vi "Set_CTRE_Status_Period.vi"(8 "error in (no error)":errorcluster, 10 "Input":T2 {"Frame" items=["Status_1_General"=5120, "Status_2_Feedback0"=5184, "Status_3_Quadrature"=5248, "Status_4_AinTempVbat"=5312, "Status_6_Misc"=5440, "Status_7_CommStatus"=5504, "Status_8_PulseWidth"=5568, "Status_9_MotProfBuffer"=5632, "Status_10_MotionMagic"=5696, "Status_11_UartGadgeteer"=5760, "Status_12_Feedback1"=5824, "Status_13_Base_PIDF0"=5888, "Status_14_Turn_PIDF1"=5952, "Status_15_FirmwareApiStatus"=6016, "Status_Brushless_Current"=4672]}, 11 "PhoenixMotorControlDevRef":T3={"DeviceStatus"={"status"=FALSE, "code"=0, "source"=""}, "Type"=enum."PWM", "PWM"={"PWM Channel"=enum."PWM 1", "DeadBand"={"Name"="", "maxPositivePwm"=0, "minPositivePwm"=0, "centerPwm"=0, "maxNegativePwm"=0, "minNegativePwm"=0, "angularRange"=0}}, "CAN"={"Device Number"=0, "SetOutput VI Ref"=variant(enum8{"Percent VBus", "Current", "Speed", "Position", "Voltage"} enum."Percent VBus"), "GetOutput VI Ref"=variant(refnum<k1> refnum), "Enable VI Ref"=variant(dbl 12.0), "Disable VI Ref"=variant(enum8{"Percent VBus", "Speed", "Position", "Slave", "Unchanged / Invalid", "Voltage Compensation", "Current", "Motion Profile"} enum."Percent VBus"), "Data"=variant}, "Invert"=FALSE, "DIO PWM"={"PWM \"Enable\" Channel"=enum."Invalid", "DIOChannel"=enum."Invalid", "PWM Rate"=0.0}}) -> (0 "error out":errorcluster, 3 "PhoenixMotorControlDevRef 2":T3={"DeviceStatus"={"status"=FALSE, "code"=0, "source"=""}, "Type"=enum."PWM", "PWM"={"PWM Channel"=enum."PWM 1", "DeadBand"={"Name"="", "maxPositivePwm"=0, "minPositivePwm"=0, "centerPwm"=0, "maxNegativePwm"=0, "minNegativePwm"=0, "angularRange"=0}}, "CAN"={"Device Number"=0, "SetOutput VI Ref"=variant(enum8{"Percent VBus", "Current", "Speed", "Position", "Voltage"} enum."Percent VBus"), "GetOutput VI Ref"=variant(refnum<k1> refnum), "Enable VI Ref"=variant(dbl 12.0), "Disable VI Ref"=variant(enum8{"Percent VBus", "Speed", "Position", "Slave", "Unchanged / Invalid", "Voltage Compensation", "Current", "Motion Profile"} enum."Percent VBus"), "Data"=variant}, "Invert"=FALSE, "DIO PWM"={"PWM \"Enable\" Channel"=enum."Invalid", "DIOChannel"=enum."Invalid", "PWM Rate"=0.0}})   [LabVIEW 2020]
uses:
  <vilib>/Rock Robotics/WPI/MotorControl/WPI_MotorControlDeviceRef.ctl
  <vilib>/Rock Robotics/WPI/MotorControl/WPI_MotorControlType.ctl
  <vilib>/Rock Robotics/SystemInterfaces/DIO/FPGA_DIOPWMChannel.ctl
  <vilib>/Rock Robotics/WPI/PWM/WPI_PWMDeadband.ctl
  <vilib>/Rock Robotics/SystemInterfaces/DIO/FPGA_DIOChannel.ctl
  <vilib>/Rock Robotics/WPI/ThirdParty/Phoenix-LabVIEW/Motor Controller/Controls/CTRE_Phoenix_MotorControl_StatusFrameEnhanced.ctl
  8bffcf12-d87b-4679-b93c-e69f5877cc70.vi
  <vilib>/Comparison/Equal/Equal Functor/Equal Functor.lvclass
panel:
  in  "High STATUS_Period(ms)":i32=10
  in  "Medium STATUS_Period(ms)":i32=50
  in  "Low STATUS_Period(ms)":i32=240
  in  "Status Frame Enum":T1=5120 items=["Status_1_General"=5120, "Status_2_Feedback0"=5184, "Status_3_Quadrature"=5248, "Status_4_AinTempVbat"=5312, "Status_6_Misc"=5440, "Status_7_CommStatus"=5504, "Status_8_PulseWidth"=5568, "Status_9_MotProfBuffer"=5632, "Status_10_MotionMagic"=5696, "Status_11_UartGadgeteer"=5760, "Status_12_Feedback1"=5824, "Status_13_Base_PIDF0"=5888, "Status_14_Turn_PIDF1"=5952, "Status_15_FirmwareApiStatus"=6016, "Status_Brushless_Current"=4672]
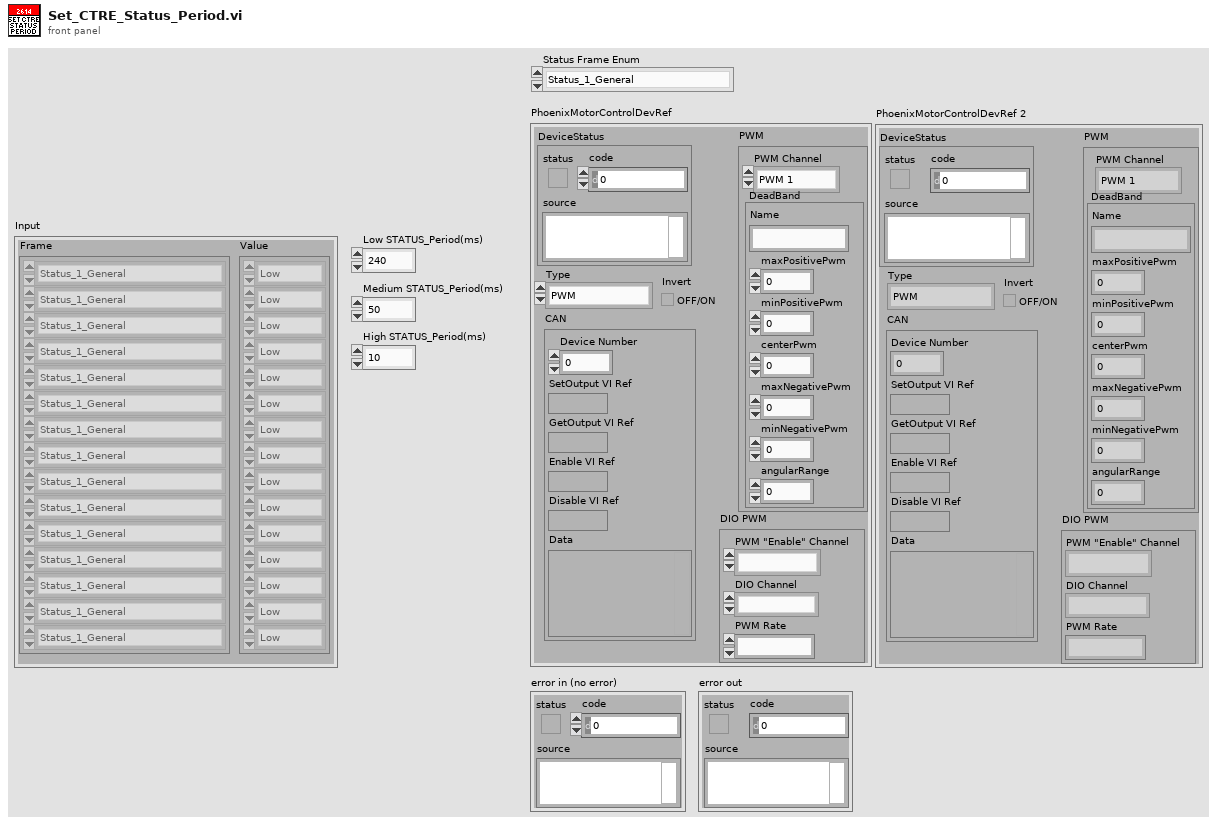
[diagram p1: front panel]
types:
  T1 = typedef "CTRE_Phoenix_MotorControl_StatusFrameEnhanced.ctl" = u16
  T2 = cluster{"Frame":T1[], "Value":enum16{"Low", "Medium", "High"}[]}
  T3 = typedef "WPI_MotorControlDeviceRef.ctl" = cluster{"DeviceStatus":errorcluster, "Type":T4, "PWM":cluster{"PWM Channel":T5, "DeadBand":T6}, "CAN":cluster{"Device Number":u8, "SetOutput VI Ref":variant, "GetOutput VI Ref":variant, "Enable VI Ref":variant, "Disable VI Ref":variant, "Data":variant}, "Invert":bool, "DIO PWM":cluster{"PWM \"Enable\" Channel":T5, "DIOChannel":T7, "PWM Rate":dbl}}
  T4 = typedef "WPI_MotorControlType.ctl" = enum16{"PWM", "CAN", "DIO PWM"}
  T5 = typedef "FPGA_DIOPWMChannel.ctl" = enum8{"PWM 0", "PWM 1", "PWM 2", "PWM 3", "PWM 4", "PWM 5", "PWM 6", "PWM 7", "PWM 8", "PWM 9", "PWM MXP 0", "PWM MXP 1", "PWM MXP 2", "PWM MXP 3", "PWM MXP 4", "PWM MXP 5", "PWM MXP 6", "PWM MXP 7", "PWM MXP 8", "PWM MXP 9", "Invalid"}
  T6 = typedef "WPI_PWMDeadband.ctl" = cluster{"Name":string, "maxPositivePwm":i32, "minPositivePwm":i32, "centerPwm":i32, "maxNegativePwm":i32, "minNegativePwm":i32, "angularRange":u16}
  T7 = typedef "FPGA_DIOChannel.ctl" = enum8{"DIO 0", "DIO 1", "DIO 2", "DIO 3", "DIO 4", "DIO 5", "DIO 6", "DIO 7", "DIO 8", "DIO 9", "DIO MXP 0", "DIO MXP 1", "DIO MXP 2", "DIO MXP 3", "DIO MXP 4", "DIO MXP 5", "DIO MXP 6", "DIO MXP 7", "DIO MXP 8", "DIO MXP 9", "DIO MXP 10", "DIO MXP 11", "DIO MXP 12", "DIO MXP 13", "DIO MXP 14", "DIO MXP 15", "SPI Port CS1", "SPI Port CS2", "SPI Port CS3", "SPI Port MISO", "SPI Port MOSI", "Invalid"}
  T8 = typedef "LVStringsAndValuesArrayTypeDef_U16.ctl" = cluster{"String":string, "Value":u16}[]
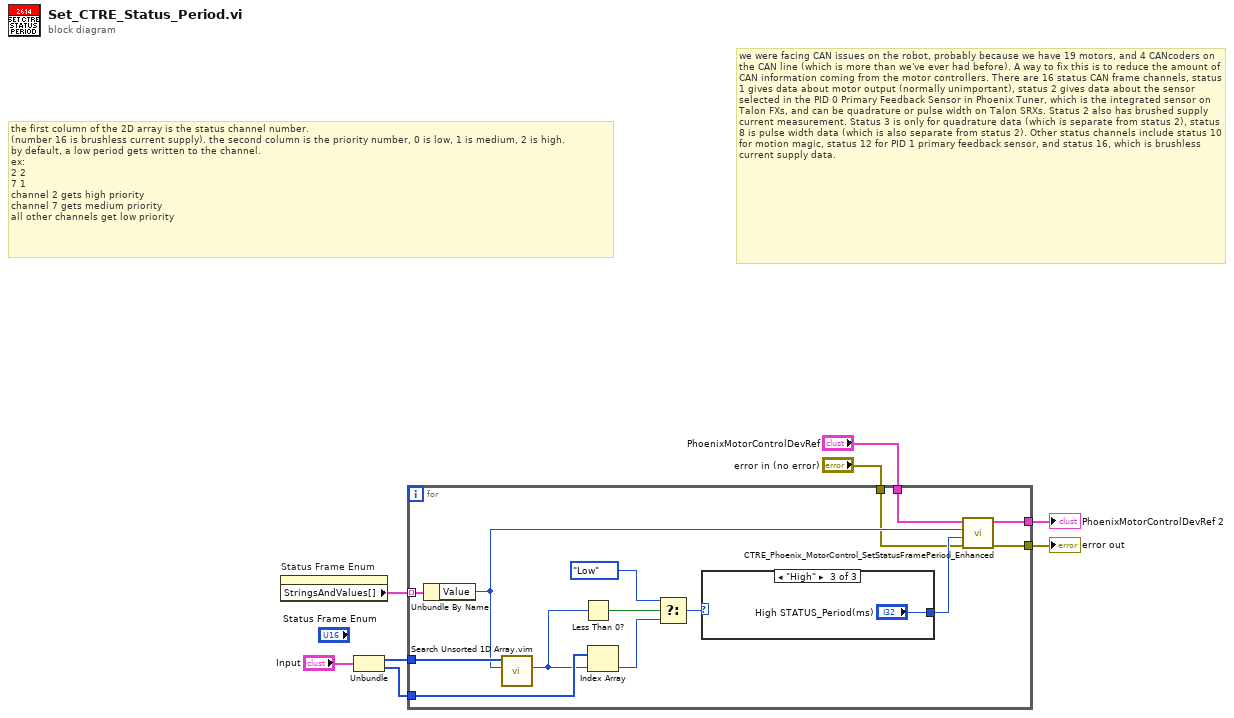
[diagram p0: block diagram]
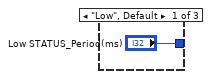
[diagram p2: hidden frame]
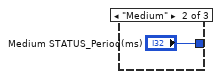
[diagram p3: hidden frame]
diagram:
  # "the first column of the 2D array is the status channel number.\n(number 16 is brushless current supply). the second column is the priority number, 0 is low, 1 is medium, 2 is high.\nby default, a low period gets written to the channel.\nex:\n2 2\n7 1\nchannel 2 gets high priority\nchannel 7 gets medium priority\nall other channels get low priority"
  # "we were facing CAN issues on the robot, probably because we have 19 motors, and 4 CANcoders on the CAN line (which is more than we've ever had before). A way to fix this is to reduce the amount of CAN information coming from the motor controllers. There are 16 status CAN frame channels, status 1 gives data about motor output (normally unimportant), status 2 gives data about the sensor selected in the PID 0 Primary Feedback Sensor in Phoenix Tuner, which is the integrated sensor on Talon FXs, and can be quadrature or pulse width on Talon SRXs. Status 2 also has brushed supply current measurement. Status 3 is only for quadrature data (which is separate from status 2), status 8 is pulse width data (which is also separate from status 2). Other status channels include status 10 for motion magic, status 12 for PID 1 primary feedback sensor, and status 16, which is brushless current supply data."
  n1 = property on="Status Frame Enum" class="Ring (strict)"() -> ("StringsAndValues[]"=w6:T8)  [unwired: 2 in, 2 out]
  n2 = Unbundle("Input") -> ("Frame"=w4:T1[], "Value"=w3:enum16{"Low", "Medium", "High"}[])
  n3 = for {
    tunnel: [w21] -> w8
    tunnel: [w20] -> w7
    tunnel: w6 -> [w12] mode=indexing
    tunnel: w4 -> [w19]
    tunnel: w3 -> [w18]
    tunnel: "error in (no error)" -> [w10]
    tunnel: "PhoenixMotorControlDevRef" -> [w9]
    n4 = Unbundle By Name(w12) -> ("Value"=w11:u16)
    n5 = call "Search Unsorted 1D Array.vim"("element"=w11, "unsorted 1D array"=w19) -> ("index of element"=w17:i32)  [unwired: 9 in]
    n6 = Less Than 0?(x=w17) -> (x < 0?=w16:bool)
    n7 = Index Array(array=w18, index=w17) -> (element=w15:enum16{"Low", "Medium", "High"})
    n8 = Select(t=enum16{"Low", "Medium", "High"}."Low", s=w16, f=w15) -> (s? t:f=w13:enum16{"Low", "Medium", "High"})
    n9 = case shown="\"High\"" w13 {
      tunnel: ["Low STATUS_Period(ms)" "Medium STATUS_Period(ms)" "High STATUS_Period(ms)"] -> w22
      frame "Low", Default {
      }
      frame "Medium" {
      }
      frame "High" {
      }
    }
    n10 = call <vilib>:"CTRE_Phoenix_MotorControl_SetStatusFramePeriod_Enhanced.vi"("error in (no error)"=w10, "periodMs"=w22, "Status Frame"=w11, "PhoenixMotorControlDevRef"=w9) -> ("error out"=w20:errorcluster, "PhoenixMotorControlDevRef"=w21:T3)  [unwired: 6 in]
  }
  "error out" <- w7
  "PhoenixMotorControlDevRef 2" <- w8
